vi "Auton Scripting.vi"   [LabVIEW 2014]
uses:
  Begin/Global Variables.vi
  <vilib>/Rock Robotics/Network Tables/SD Read Boolean.vi
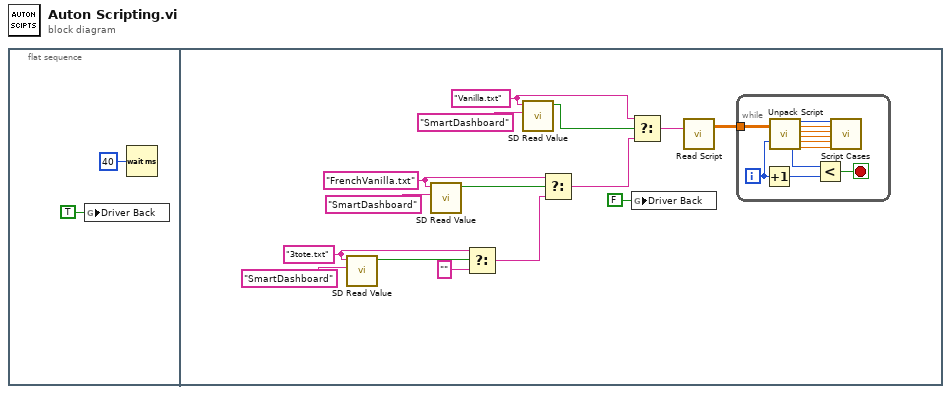
[diagram p0: block diagram]
diagram:
  n1 = flat-sequence {
    frame #0 {
      n2 = global write "Global Variables.vi" "Driver Back"(TRUE ("Driver Back")) -> ()
      n3 = Wait (ms)(milliseconds to wait=u32 40) -> ()  [unwired: 1 out]
    }
    frame #1 {
      w5 = "3tote.txt" ("Name")
      w8 = "FrenchVanilla.txt" ("Name")
      w10 = "Vanilla.txt" ("Name")
      n4 = call-poly <vilib>:"SD Read Value.vi"("Table Prefix"="SmartDashboard", "Name"=w5) -> ("Boolean"=w6:bool)  [unwired: 7 in, 2 out]
      n5 = call-poly <vilib>:"SD Read Value.vi"("Table Prefix"="SmartDashboard", "Name"=w8) -> ("Boolean"=w7:bool)  [unwired: 7 in, 2 out]
      n6 = Select(t=w5, s=w6, f="") -> (s? t:f=w4:string)
      n7 = call-poly <vilib>:"SD Read Value.vi"("Table Prefix"="SmartDashboard", "Name"=w10) -> ("Boolean"=w12:bool)  [unwired: 7 in, 2 out]
      n8 = Select(t=w8, s=w7, f=w4) -> (s? t:f=w9:string)
      n9 = Select(t=w10, s=w12, f=w9) -> (s? t:f=w11:string)
      n10 = global write "Global Variables.vi" "Driver Back"(FALSE ("Driver Back")) -> ()
      n11 = call "Read Script.vi"("script name"=w11) -> ("output array"=w17:dbl[][])  [unwired: 1 in, 1 out]
      n12 = while {
        tunnel: w17 -> [w28]
        i -> [w21]
        stop <- w18 stop-if-true
        n13 = Increment(x=w21) -> (x+1=w19:i32)
        n14 = call "Unpack Script.vi"("script"=w28, "index"=w21) -> ("# of primitives"=w20:i32, "primitive"=w27:i32, "argument 1"=w26:dbl, "argument 2"=w25:dbl, "argument 3"=w24:dbl, "argument 4"=w23:dbl, "argument 5"=w22:dbl)  [unwired: 11 in]
        n15 = Less?(x=w20, y=w19) -> (x < y?=w18:bool)
        n16 = call "Script Cases.vi"("primitive"=w27, "argument 1"=w26, "argument 2"=w25, "argument 3"=w24, "argument 4"=w23, "argument 5"=w22) -> ()  [unwired: 14 in]
      }
    }
  }
